vi "Add Request.vi"(5 "HTTPS?":bool, 7 "Request":refnum<class "Request.lvclass">, 10 "error in (no error)":errorcluster, 11 "RequestTraceLog in":refnum<class "RequestTraceLog.lvclass">) -> (2 "error out":errorcluster, 3 "RequestTraceLog out":refnum<class "RequestTraceLog.lvclass">)   [LabVIEW 2020, in "HTTP Server.lvlib" / "RequestTraceLog.lvclass"]
uses:
  RequestTraceLog.lvclass
  lv-http-util/HTTP Utils/Request/Request.lvclass
  RequestTraceLog.lvclass/RequestTraceLog.ctl
  lv-uri/URI/URI/URI.lvclass
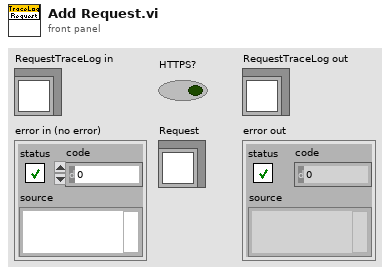
[diagram p1: front panel]
types:
  T1 = typedef "HTTP Utils.lvlib/Method.ctl" = enum16{"GET", "HEAD", "POST", "PUT", "DELETE", "CONNECT", "OPTIONS", "TRACE", "PATCH"}
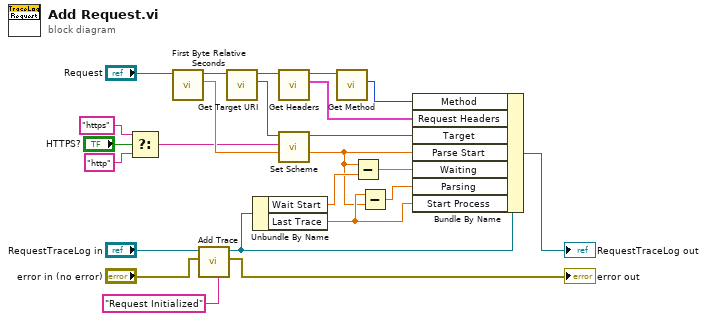
[diagram p0: block diagram]
diagram:
  n1 = Select(t="https", s="HTTPS?", f="http") -> (s? t:f=w1:string)
  n2 = call "First Byte Relative Seconds.vi"("Request in"="Request") -> ("First Byte Relative Seconds"=w9:dbl, "Request out"=w14:refnum<class "Request.lvclass">)  [unwired: 8 in, 1 out]
  n3 = call "Add Trace.vi"("Info"="Request Initialized", "error in (no error)"="error in (no error)", "RequestTraceLog in"="RequestTraceLog in") -> ("error out"=→"error out":errorcluster, "RequestTraceLog out"=w18:refnum<class "RequestTraceLog.lvclass">)  [unwired: 7 in]
  n4 = call "Get Target URI.vi"("Request in"=w14) -> ("Target URI"=w2:refnum<class "URI.lvclass">, "Request out"=w17:refnum<class "Request.lvclass">)  [unwired: 8 in, 1 out]
  n5 = Unbundle By Name(w18) -> ("Wait Start"=w12:dbl, "Last Trace"=w11:dbl)
  n6 = call "Get Headers.vi"("Request in"=w17) -> ("Headers"=w16:cluster{"Header":string, "Value":string}[], "Request out"=w8:refnum<class "Request.lvclass">)  [unwired: 8 in, 1 out]
  n7 = call "Set Scheme.vi"("Scheme"=w1, "URI in"=w2) -> ("URI out"=w3:refnum<class "URI.lvclass">)  [unwired: 9 in]
  n8 = call "Get Method.vi"("Request in"=w8) -> ("Method"=w7:T1)  [unwired: 8 in, 2 out]
  n9 = Subtract(x=w9, y=w12) -> (x-y=w13:dbl)
  n10 = Subtract(x=w11, y=w9) -> (x-y=w10:dbl)
  n11 = Bundle By Name(cluster=w18, "Method"=w7, "Request Headers"=w16, "Target"=w3, "Parse Start"=w9, "Waiting"=w13, "Parsing"=w10, "Start Process"=w11) -> (→"RequestTraceLog out":refnum<class "RequestTraceLog.lvclass">)
